vi "Get Angle Offset File Path.vi"(11 "servo ID (0)":i32) -> (3 "angle offset file path":path)   [LabVIEW 2017, in "NI_Robotics_Starter Kit Servo Motor.lvclass"]
uses:
  <vilib>/robotics/Starter Kit/Servo Motor/NI_Robotics_Starter Kit Servo Motor.lvclass
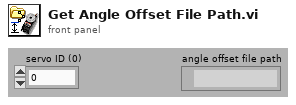
[diagram p1: front panel]
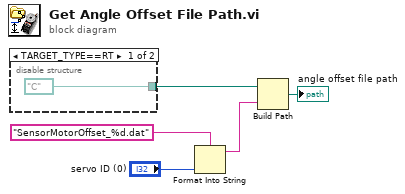
[diagram p0: block diagram]
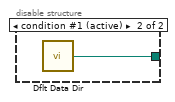
[diagram p2: hidden frame]
diagram:
  n1 = disable-structure shown="TARGET_TYPE==RT" {
    disable-tunnel: [path "C:/" ("file path (use dialog)") w7] -> w2
    frame condition #0 {
    }
    frame condition #1 (active) {
      n2 = call <vilib>:"Dflt Data Dir.vi"() -> ("App:Default Data Directory"=w7:path)
    }
  }
  n3 = Format Into String(format string="SensorMotorOffset_%d.dat", "servo ID (0)") -> (resulting string=w5:string)  [unwired: 2 in, 1 out]
  n4 = Build Path(base path=w2, name or relative path=w5) -> (appended path=→"angle offset file path":path)
